vi "Ramping.vi"(10 "Get Motor":dbl, 11 "Wanted Motor Value":dbl) -> (3 "Current Motor Value":dbl)   [LabVIEW 2012]
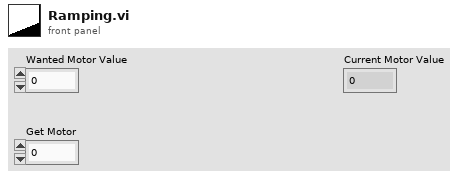
[diagram p1: front panel]
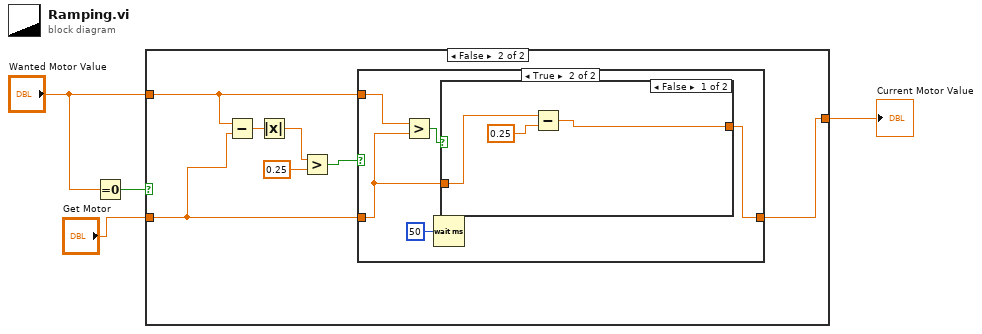
[diagram p0: block diagram]
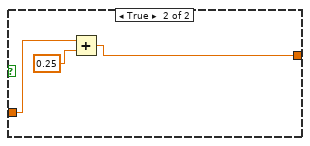
[diagram p4: hidden frame]
diagram:
  n1 = Equal To 0?(x="Wanted Motor Value") -> (x = 0?=w3:bool)
  n2 = case shown="False" w3 {
    tunnel: "Wanted Motor Value" -> [w5 w7]
    tunnel: [w5 w8] -> w2
    tunnel: "Get Motor" -> [_ w9]
    frame True {
    }
    frame False {
      n3 = Subtract(x=w7, y=w9) -> (x-y=w12:dbl)
      n4 = Absolute Value(x=w12) -> (abs(x)=w11:dbl)
      n5 = Greater?(x=w11, y=0.25) -> (0:w6:bool)
      n6 = case shown="True" w6 {
        tunnel: w9 -> [_ w14]
        tunnel: [w13 w18] -> w8
        tunnel: w7 -> [w13 w17]
        frame False {
        }
        frame True {
          n7 = Greater?(x=w17, y=w14) -> (0:w16:bool)
          n8 = Wait (ms)(milliseconds to wait=u32 50) -> ()  [unwired: 1 out]
          n9 = case shown="False" w16 {
            tunnel: w14 -> [w21 w24]
            tunnel: [w19 w22] -> w18
            frame False {
              n10 = Subtract(x=w21, y=0.25) -> (x-y=w19:dbl)
            }
            frame True {
              n11 = Add(x=w24, y=0.25) -> (x+y=w22:dbl)
            }
          }
        }
      }
    }
  }
  "Current Motor Value" <- w2
